vi "AxesWindow.vi"(0 "System no.":i32=1 min=1 step=1, 5 "error in":errorcluster) -> (19 "error out":errorcluster)   [LabVIEW 2014]
doc: "This VI allows the user to enable or disable the servo or to perform a reference move of the selectet axes.\nSelecting \"Cancel FRF\" or pressing the Escape key will stop the reference motion of all axes by sending a \"#24\" command to the controller.\nThis VI opens modal so that the communication, especially the STOP command, is not disturbed by any other processes."
uses:
  C:/ProgramData/PI/LabVIEW/Low Level/General command.llb/Global2 (Array).vi
  C:/ProgramData/PI/LabVIEW/Low Level/Support.llb/HasCommandArray?.vi
panel:
  in  "Cancel FRF":bool
  in  "Stop":bool
  in  "Axes status":T1(array[cluster])
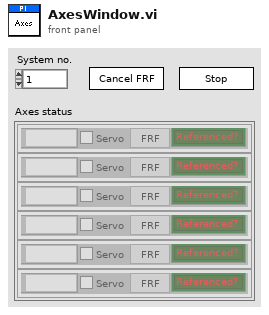
[diagram p1: front panel]
types:
  T1 = cluster{"FRF":bool, "Servo":bool, "Referenced?":bool, "Axis name":string}[]
  T2 = cluster{"FRF":bool, "Servo":bool, "Referenced?":bool, "Axis name":string}
  T3 = typedef "Controller names.ctl" = enum16{"None", "Analog", "C-702", "C-413", "C-414", "C-843", "C-843.PM", "C-844", "C-848", "C-865", "C-866", "C-867", "C-877", "C-880", "C-884", "C-885", "C-886", "C-887", "C-891", "E-135", "E-516", "E-517", "E-518", "E-709", "E-710", "E-712", "E-725", "E-727", "E-753", "E-754", "E-755", "E-761", "E-816", "E-861", "E-870", "E-871", "E-872", "E-873", "E-874", "F-206", "HydraPollux", "M-840", "M-850", "M-8X0", "Mercury", "Mercury_GCS", "PI_GCS2"}
  T4 = cluster{"Conn. axes":string[], "Controller name":T3}[]
  T5 = cluster{"Conn. axes":string[], "Controller name":T3}
  T6 = cluster{"FRF":bool, "Servo":bool, "Referenced?":bool, "Axis name":bool}
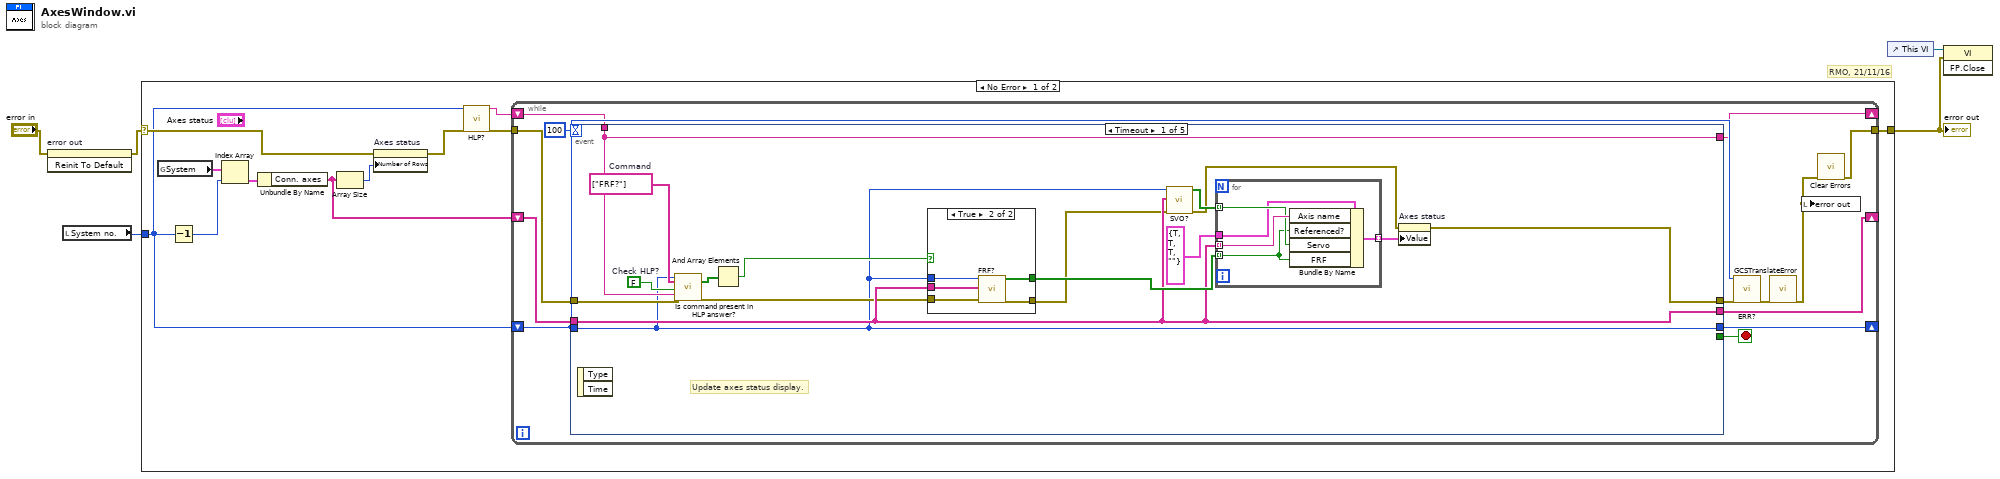
[diagram p0: block diagram]
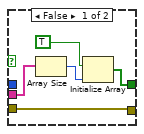
[diagram p2: hidden frame]
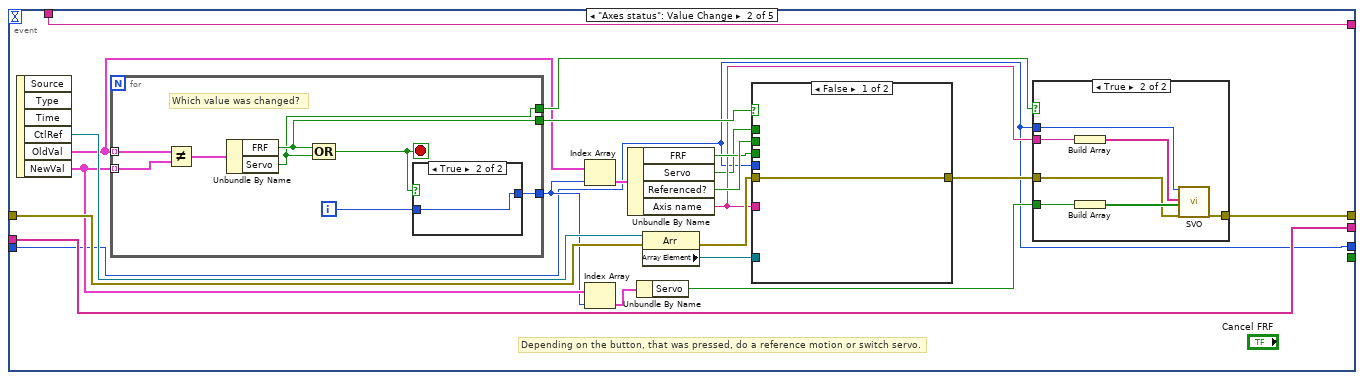
[diagram p3: hidden frame]
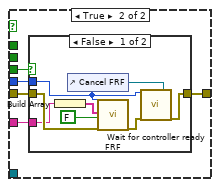
[diagram p5: hidden frame]
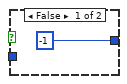
[diagram p7: hidden frame]
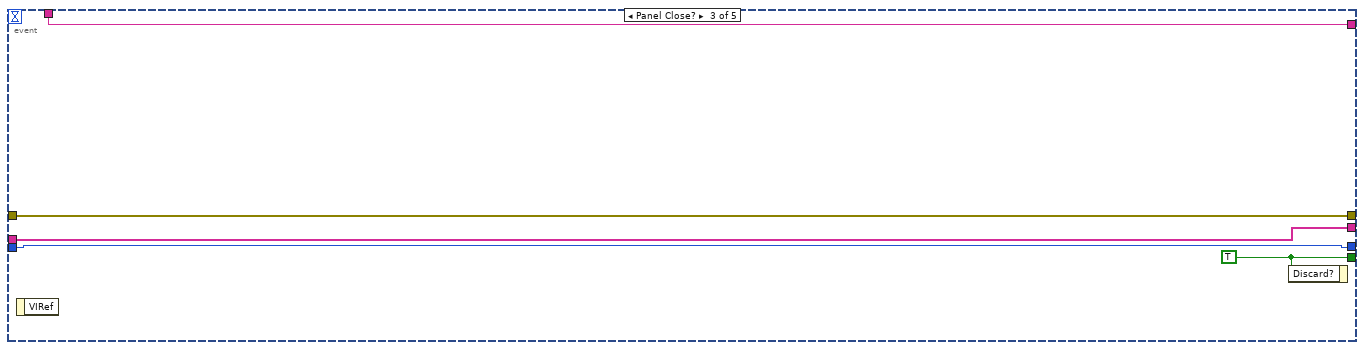
[diagram p8: hidden frame]
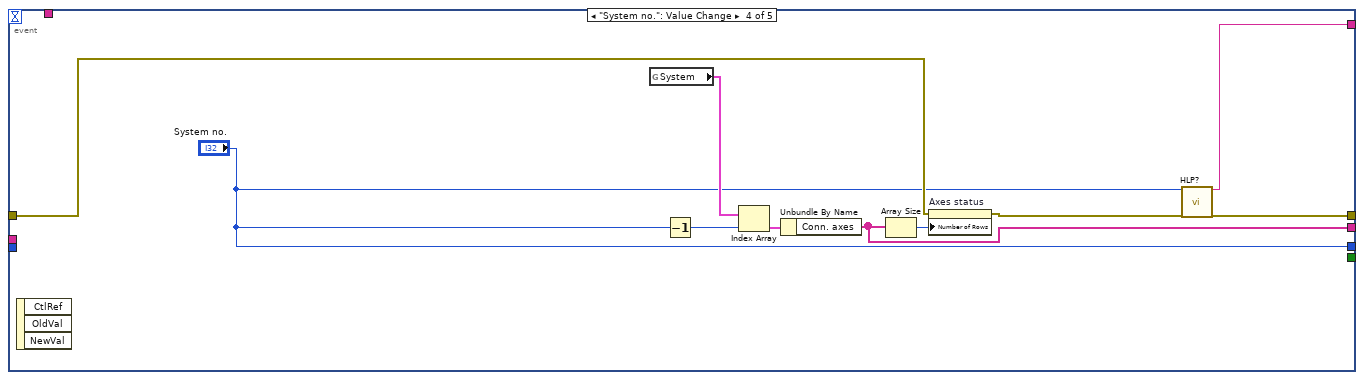
[diagram p9: hidden frame]
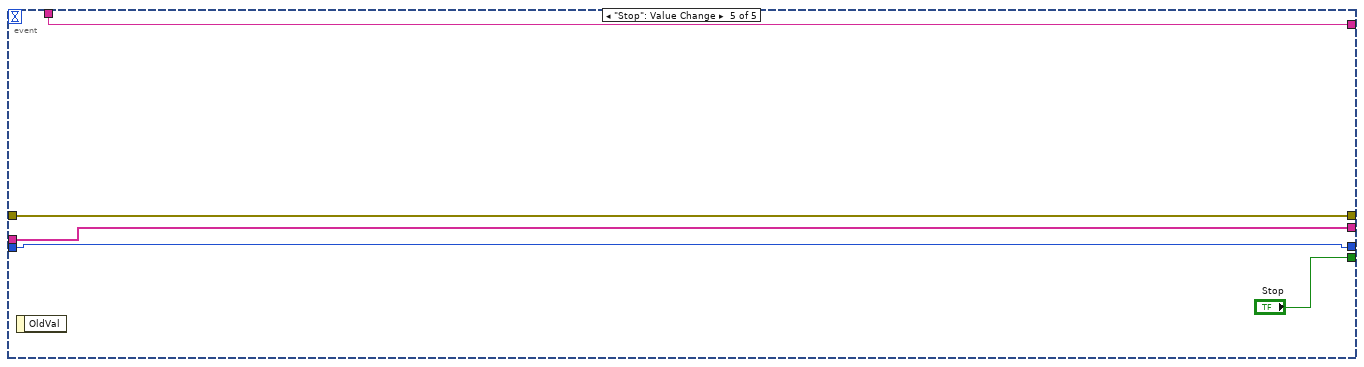
[diagram p10: hidden frame]
diagram:
  # "RMO, 21/11/16"
  n1 = invoke on="error out" class="Clust (strict)" method="Reinit To Default"(error in="error in") -> (error out=w4:errorcluster)  [unwired: 2 in, 2 out]
  n2 = local read "System no."() -> (w1:i32)
  n3 = case shown="No Error" w4 {
    selector: w4 -> [w11 w135]
    tunnel: [w10 w135] -> w2
    tunnel: w1 -> [w7 _]
    frame No Error {
      n4 = global read "Global2 (Array).vi" "System"() -> (w16:T4)
      n5 = Decrement(x=w7) -> (x-1=w15:i32)
      n6 = Index Array(array=w16, index=w15) -> (element=w14:T5)
      n7 = Unbundle By Name(w14) -> ("Conn. axes"=w12:string[])
      n8 = Array Size(array=w12) -> (size(s)=w13:i32)
      n9 = property on="Axes status" class="Arr"(error in=w11, "Number of Rows"=w13) -> (error out=w9:errorcluster)  [unwired: 1 in, 1 out]
      n10 = call "HLP?.vi"("System no."=w7, "error in"=w9) -> ("Help string"=w6:string, "error out"=w8:errorcluster)  [unwired: 16 out]
      n11 = while {
        shift-right: [w20] -> _
        shift-left: w12 -> [w29]
        tunnel: w8 -> [w28]
        tunnel: [w22] -> w10
        shift-right: [w19] -> _
        shift-left: w6 -> [w18]
        shift-right: [w17] -> _
        shift-left: w7 -> [w23]
        stop <- w27 stop-if-true
        n12 = event shown="[0] Timeout" {
          selector: _ -> [_ _ _ _ _]
          dyn-events: _ -> [_ _ _ _ _]
          timeout: 100 -> [_ _ _ _ _]
          tunnel: w29 -> [w39 w66 w117 _ w132]
          tunnel: w28 -> [w36 w80 w118 w125 w133]
          tunnel: [w41 w67 w118 w122 w133] -> w25
          tunnel: [_ _ w119 _ "Stop"] -> w27
          tunnel: w23 -> [w30 w61 w115 _ w130]
          tunnel: [w39 w66 w117 w124 w132] -> w20
          tunnel: [w37 w62 w116 w121 w131] -> w19
          tunnel: w18 -> [w37 w62 w116 _ w131]
          tunnel: [w30 w61 w115 "System no." w130] -> w17
          event Timeout {
            w34 = string[] ["FRF?"]  # Command
            w35 = FALSE  # Check HLP?
            # "Update axes status display."
            n13 = event-data() -> ()  [unwired: 3 out]
            n14 = call-poly "Is command present in HLP answer?.vi"("System no."=w30, "Command"=w34, "Check HLP?"=w35, "HLP? answer"=w37, "error in"=w36) -> ("Is command available?"=w33:bool[], "error out"=w32:errorcluster)  [unwired: 12 in, 1 out]
            n15 = And Array Elements(Boolean array=w33) -> (logical AND=w31:bool)
            n16 = case shown="True" w31 {
              tunnel: [w46 w55] -> w44
              tunnel: w39 -> [w49 w54]
              tunnel: [w50 w53] -> w38
              tunnel: w30 -> [_ w52]
              tunnel: w32 -> [w50 w51]
              frame False {
                n17 = Array Size(array=w49) -> (size(s)=w47:i32)
                n18 = Initialize Array(TRUE, w47) -> (w46:bool[])
              }
              frame True {
                n19 = call "FRF?.vi"("System no."=w52, "Axes to query"=w54, "error in"=w51) -> ("Referenced?"=w55:bool[], "error out"=w53:errorcluster)  [unwired: 2 in, 13 out]
              }
            }
            n20 = call "SVO?.vi"("System no."=w30, "Axes to query"=w39, "error in"=w38) -> ("Servo status?"=w45:bool[], "error out"=w42:errorcluster)  [unwired: 2 in, 13 out]
            n21 = for {
              tunnel: w39 -> [w60] mode=indexing
              tunnel: [w59] -> w40 mode=indexing
              tunnel: w45 -> [w58] mode=indexing
              tunnel: w44 -> [w57] mode=indexing
              tunnel: T2 {"FRF"=TRUE, "Servo"=TRUE, "Referenced?"=TRUE, "Axis name"=""} ("Axis status") -> [w56]
              n22 = Bundle By Name(cluster=w56, "Axis name"=w60, "Referenced?"=w57, "Servo"=w58, "FRF"=w57) -> (w59:T2)
            }
            n23 = property on="Axes status" class="Arr"(error in=w42, "Value"=w40) -> (error out=w41:errorcluster)  [unwired: 1 in, 1 out]
          }
          event "Axes status": Value Change {
            # "Depending on the button, that was pressed, do a reference motion or switch servo."
            n24 = event-data() -> ("CtlRef"=w81:refnum<vi>, "OldVal"=w63:T1, "NewVal"=w70:T1)  [unwired: 4 out]
            n25 = for {
              tunnel: w63 -> [w112] mode=indexing
              tunnel: w70 -> [w111] mode=indexing
              tunnel: [w108] -> w65
              tunnel: [w106] -> w76
              tunnel: [w105] -> w74
              i -> [w109]
              stop <- w107 stop-if-true
              # "Which value was changed?"
              n26 = Not Equal?(x=w112, y=w111) -> (x != y?=w110:T6)
              n27 = Unbundle By Name(w110) -> ("FRF"=w106:bool, "Servo"=w105:bool)
              n28 = Compound Arithmetic op=OR(w106, w105) -> (w107:bool)
              n29 = case shown="True" w107 {
                tunnel: w109 -> [_ w114]
                tunnel: [-1 w114] -> w108
                frame False {
                }
                frame True {
                }
              }
            }
            n30 = Index Array(array=w63, index=w65) -> (element=w64:T2)
            n31 = Index Array(array=w70, index=w65) -> (element=w69:T2)
            n32 = Unbundle By Name(w64) -> ("FRF"=w75:bool, "Servo"=w71:bool, "Referenced?"=w77:bool, "Axis name"=w72:string)
            n33 = Unbundle By Name(w69) -> ("Servo"=w68:bool)
            n34 = property class="Arr"(reference=w81, error in=w80) -> (error out=w78:errorcluster, "Array Element"=w79:refnum<vi>)  [unwired: 1 out]
            n35 = case shown="False" w76 {
              tunnel: w79 -> [_ _]
              tunnel: w78 -> [w90 w95]
              tunnel: [w90 w91] -> w73
              tunnel: w71 -> [_ _]
              tunnel: w77 -> [_ _]
              tunnel: w72 -> [_ w92]
              tunnel: w75 -> [_ w94]
              tunnel: w61 -> [_ w93]
              frame False {
              }
              frame True {
                n36 = case shown="False" w94 {
                  tunnel: w95 -> [w102 w104]
                  tunnel: [w101 w104] -> w91
                  tunnel: w93 -> [w100 _]
                  tunnel: w92 -> [w96 _]
                  frame False {
                    n37 = Build Array(w96) -> (w103:string[])
                    n38 = control-ref of="Cancel FRF"() -> (w97:refnum<vi>)
                    n39 = call "FRF.vi"("System no."=w100, "Affected axes"=w103, "All axes?"=FALSE, "error in"=w102) -> ("error out"=w98:errorcluster)  [unwired: 1 in, 14 out]
                    n40 = call "Wait for controller ready.vi"("System no."=w100, "error in"=w98, "Stop refnum"=w97) -> ("error out"=w101:errorcluster)  [unwired: 1 in, 15 out]
                  }
                  frame True {
                  }
                }
              }
            }
            n41 = case shown="True" w74 {
              tunnel: w73 -> [w82 w84]
              tunnel: [w82 w83] -> w67
              tunnel: w61 -> [_ w89]
              tunnel: w72 -> [_ w88]
              tunnel: w68 -> [_ w86]
              frame False {
              }
              frame True {
                n42 = Build Array(w88) -> (w87:string[])
                n43 = Build Array(w86) -> (w85:bool[])
                n44 = call "SVO.vi"("System no."=w89, "Axes to command"=w87, "Servo mode"=w85, "error in"=w84) -> ("error out"=w83:errorcluster)  [unwired: 1 in, 14 out]
              }
            }
          }
          event Panel Close? {
            w119 = TRUE
            n45 = event-data() -> ()  [unwired: 2 out]
            n46 = event-data("Discard?"=w119) -> ()  [unwired: 1 in, 1 out]
          }
          event "System no.": Value Change {
            n47 = event-data() -> ()  [unwired: 4 out]
            n48 = global read "Global2 (Array).vi" "System"() -> (w127:T4)
            n49 = Decrement(x="System no.") -> (x-1=w128:i32)
            n50 = Index Array(array=w127, index=w128) -> (element=w129:T5)
            n51 = Unbundle By Name(w129) -> ("Conn. axes"=w124:string[])
            n52 = Array Size(array=w124) -> (size(s)=w126:i32)
            n53 = property on="Axes status" class="Arr"(error in=w125, "Number of Rows"=w126) -> (error out=w123:errorcluster)  [unwired: 1 in, 1 out]
            n54 = call "HLP?.vi"("System no."="System no.", "error in"=w123) -> ("Help string"=w121:string, "error out"=w122:errorcluster)  [unwired: 16 out]
          }
          event "Stop": Value Change {
            n55 = event-data() -> ()  [unwired: 2 out]
          }
        }
        n56 = call "ERR?.vi"("System no."=w23, "error in"=w25) -> ("error out"=w24:errorcluster)  [unwired: 17 out]
        n57 = call "GCSTranslateError.vi"("error in"=w24) -> ("error out"=w21:errorcluster)  [unwired: 18 out]
        n58 = local write "error out"(w21) -> ()
        n59 = call <vilib>:"Clear Errors.vi"("error in (no error)"=w21) -> ("error out"=w22:errorcluster)  [unwired: 1 in, 5 out]
      }
    }
    frame Error {
    }
  }
  "error out" <- w2
  n60 = control-ref of="This VI"() -> (w3:refnum<vi>)
  n61 = invoke class="VI" method="FP.Close"(reference=w3, error in=w2) -> ()  [unwired: 1 in, 3 out]
